vi "PositionControl.vi"(7 "Mode":T1=enum."Read Pos", 8 "error in (no error)":errorcluster, 9 "Calibration":cluster{dbl, "MicrostepMode":u32}[](array[cluster]), 10 "Move to":sgl[](array[numeric]), 11 "IDs":i32[](array[numeric])) -> (0 "error out":errorcluster, 1 "Moving?":bool, 2 "Position":sgl[](array[numeric]), 3 "Success?":bool)   [LabVIEW 2020]
uses:
  PosCtrlOptions.ctl
  libximc.lvlib
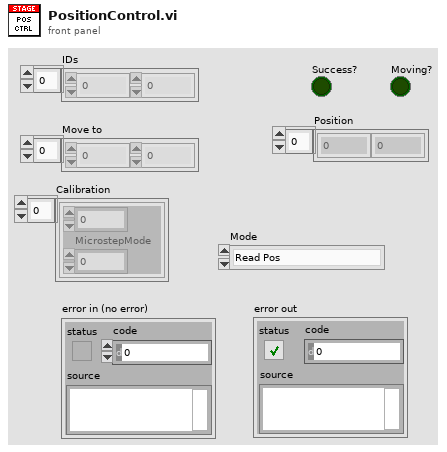
[diagram p1: front panel]
types:
  T1 = typedef "PosCtrlOptions.ctl" = enum16{"Move X", "Move Y", "Both X and Y", "Read Pos", "None"}
  T2 = cluster{"MoveSts":u32, "MvCmdSts":u32, "PWRSts":u32, "EncSts":u32, "WindSts":u32, "CurPosition":sgl, "EncPosition":i64, "CurSpeed":sgl, "Ipwr":i32, "Upwr":i32, "Iusb":i32, "Uusb":i32, "CurT":i32, "Flags":u32, "GPIOFlags":u32, "CmdBufFreeSpace":u32}
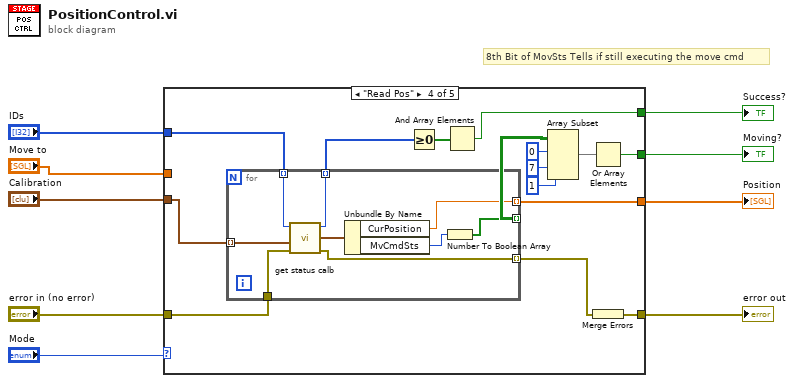
[diagram p0: block diagram]
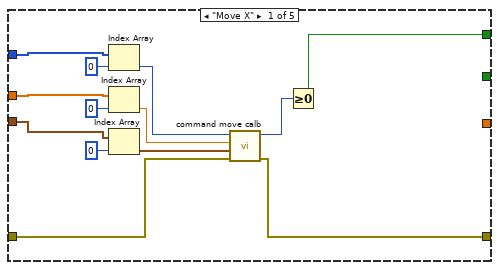
[diagram p2: hidden frame]
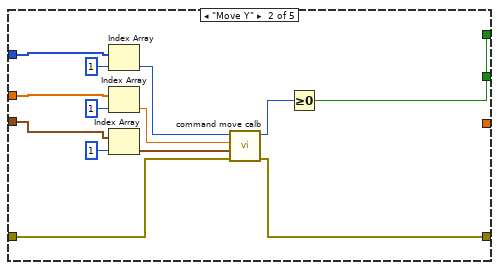
[diagram p3: hidden frame]
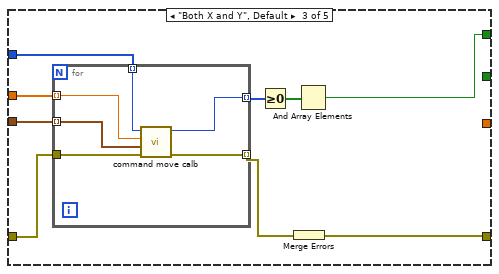
[diagram p4: hidden frame]
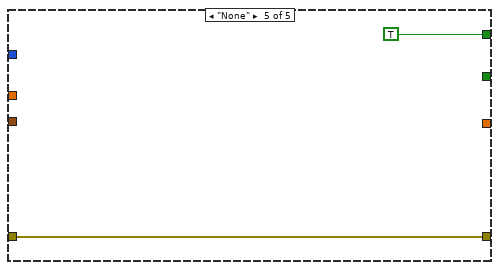
[diagram p5: hidden frame]
diagram:
  # "8th Bit of MovSts Tells if still executing the move cmd"
  n1 = case shown="\"Read Pos\"" "Mode" {
    tunnel: "Move to" -> [w18 w31 w44 _ _]
    tunnel: "IDs" -> [w22 w35 w43 w62 _]
    tunnel: "error in (no error)" -> [w13 w26 w42 w60 w76]
    tunnel: [w12 w25 w39 w59 w76] -> w4
    tunnel: "Calibration" -> [w15 w28 w40 w61 _]
    tunnel: [w10 w24 w36 w64 TRUE] -> w3
    tunnel: [_ _ _ w57 _] -> w2
    tunnel: [_ _ _ w51 _] -> w1
    frame "Move X" {
      n2 = Index Array(array=w22, index=0) -> (element=w20:i32)
      n3 = Index Array(array=w18, index=0) -> (element=w17:sgl)
      n4 = Index Array(array=w15, index=0) -> (element=w14:cluster{dbl, "MicrostepMode":u32})
      n5 = call "command move calb.vi"("error in (no error)"=w13, "calibration"=w14, "Position"=w17, "id"=w20) -> ("error out"=w12:errorcluster, "function return"=w11:i32)  [unwired: 6 in]
      n6 = Greater Or Equal To 0?(x=w11) -> (x >= 0?=w10:bool)
    }
    frame "Move Y" {
      n7 = Index Array(array=w35, index=1) -> (element=w33:i32)
      n8 = Index Array(array=w31, index=1) -> (element=w30:sgl)
      n9 = Index Array(array=w28, index=1) -> (element=w27:cluster{dbl, "MicrostepMode":u32})
      n10 = call "command move calb.vi"("error in (no error)"=w26, "calibration"=w27, "Position"=w30, "id"=w33) -> ("error out"=w25:errorcluster, "function return"=w23:i32)  [unwired: 6 in]
      n11 = Greater Or Equal To 0?(x=w23) -> (x >= 0?=w24:bool)
    }
    frame "Both X and Y", Default {
      n12 = for {
        tunnel: w44 -> [w50] mode=indexing
        tunnel: [w49] -> w41 mode=indexing
        tunnel: w43 -> [w48] mode=indexing
        tunnel: w42 -> [w47]
        tunnel: [w46] -> w37 mode=indexing
        tunnel: w40 -> [w45] mode=indexing
        n13 = call "command move calb.vi"("error in (no error)"=w47, "calibration"=w45, "Position"=w50, "id"=w48) -> ("error out"=w49:errorcluster, "function return"=w46:i32)  [unwired: 6 in]
      }
      n14 = Greater Or Equal To 0?(x=w37) -> (x >= 0?=w38:bool[])
      n15 = Merge Errors(w41) -> (w39:errorcluster)
      n16 = And Array Elements(Boolean array=w38) -> (logical AND=w36:bool)
    }
    frame "Read Pos" {
      n17 = for {
        tunnel: w62 -> [w74] mode=indexing
        tunnel: [w73] -> w58 mode=indexing
        tunnel: w60 -> [w71]
        tunnel: w61 -> [w70] mode=indexing
        tunnel: [w69] -> w57 mode=indexing
        tunnel: [w68] -> w63 mode=indexing
        tunnel: [w66] -> w52 mode=indexing
        n18 = call "get status calb.vi"("error in (no error)"=w71, "calibration"=w70, "id"=w74) -> ("error out"=w73:errorcluster, "status out"=w72:T2, "function return"=w68:i32)  [unwired: 6 in]
        n19 = Unbundle By Name(w72) -> ("CurPosition"=w69:sgl, "MvCmdSts"=w67:u32)
        n20 = Number To Boolean Array(number=w67) -> (Boolean array=w66:bool[])
      }
      n21 = Greater Or Equal To 0?(x=w63) -> (x >= 0?=w65:bool[])
      n22 = And Array Elements(Boolean array=w65) -> (logical AND=w64:bool)
      n23 = Array Subset(array=w52, index (row)=0 ("index"), index (col)=7 ("index"), length (col)=1 ("length")) -> (w53:bool[][])  [unwired: 1 in]
      n24 = Or Array Elements(Boolean array=w53) -> (logical OR=w51:bool)
      n25 = Merge Errors(w58) -> (w59:errorcluster)
    }
    frame "None" {
    }
  }
  "error out" <- w4
  "Success?" <- w3
  "Position" <- w2
  "Moving?" <- w1
